vi "Rules.vi"   [LabVIEW 2024]
panel:
  # "Rules"
  # "1. ADADAADADADDADA"
  # "2. ADADAADADADDADA"
  # "3. ADADAADADADDADA"
  # "4. ADADAADADADDADA"
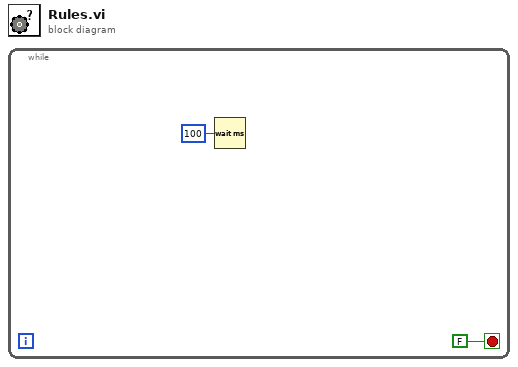
[diagram p0: block diagram]
diagram:
  n1 = while {
    stop <- FALSE stop-if-true
    n2 = Wait (ms)(milliseconds to wait=u32 100) -> ()  [unwired: 1 out]
  }
